vi "naploteszt.vi"() -> ()   [LabVIEW 2013]
panel:
  out "concatenated string 2":string
  out "concatenated string":string
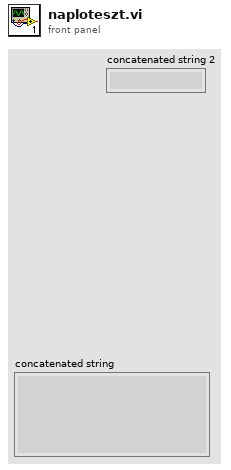
[diagram p1: front panel]
types:
  T1 = enum16{"open", "replace", "create", "open or create", "replace or create", "replace or create with confirmation"}
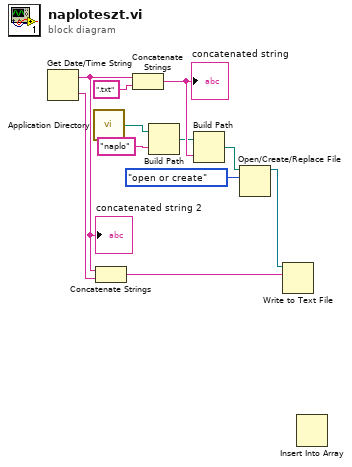
[diagram p0: block diagram]
diagram:
  n1 = Get Date/Time String() -> (date string=w3:string, time string=w2:string)  [unwired: 3 in]
  "concatenated string 2" <- w3
  n2 = call <vilib>:"Application Directory.vi"() -> ("Application Directory"=w10:path)
  n3 = Concatenate Strings(w3, w2) -> (w1:string)
  n4 = Concatenate Strings(w3, ".txt" ("name or relative path")) -> (w8:string)
  "concatenated string" <- w8
  n5 = Build Path(base path=w10, name or relative path="naplo") -> (appended path=w7:path)
  n6 = Build Path(base path=w7, name or relative path=w8) -> (appended path=w6:path)
  n7 = Open/Create/Replace File(file path (use dialog)=w6, operation (0:open)=T1."open or create") -> (refnum out=w5:refnum<file>)  [unwired: 4 in, 2 out]
  n8 = Write to Text File(file (use dialog)=w5, text=w1) -> ()  [unwired: 2 in, 3 out]
  n9 = Insert Into Array() -> ()  [unwired: 3 in, 1 out]
